vi "get jsonrpc and id values.vi"(8 "error in (no error)":errorcluster, 11 "Request":variant) -> (0 "error out":errorcluster, 1 "id":variant, 2 "jsonrpc":string)   [LabVIEW 2017, in "JSONRPC Server.lvclass"]
uses:
  JSONRPC Server.lvclass
  <vilib>/National Instruments/Variant Data Manipulation/Variant Data Manipulation.lvlib
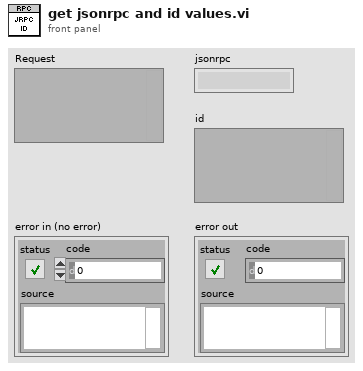
[diagram p1: front panel]
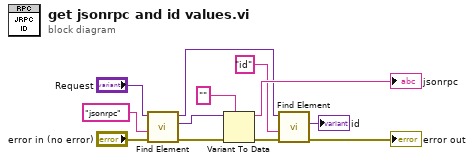
[diagram p0: block diagram]
diagram:
  n1 = call <vilib>:"Find Element.vi"("error in (no error)"="error in (no error)", "Name"="jsonrpc", "Variant (Cluster) in"="Request") -> ("error out"=w10:errorcluster, "element"=w7:variant, "Variant (Cluster) out"=w3:variant)  [unwired: 4 in, 2 out]
  n2 = Variant To Data(error in=w10, type="" ("Name"), Variant=w7) -> (data=→"jsonrpc":string, error out=w11:errorcluster)
  n3 = call <vilib>:"Find Element.vi"("error in (no error)"=w11, "Name"="id", "Variant (Cluster) in"=w3) -> ("error out"=→"error out":errorcluster, "element"=→"id":variant)  [unwired: 4 in, 3 out]
